vi "VideoWriter GetBackendName.vi"(8 "error in (no error)":errorcluster, 11 "VideoWriter in":refnum<class "VideoWriter.lvclass">) -> (0 "error out":errorcluster, 2 "BackendName":string, 3 "VideoWriter out":refnum<class "VideoWriter.lvclass">)   [LabVIEW 2020, in "OpenLvVision_OpenCv.lvlib" / "VideoWriter.lvclass"]
doc: "Returns used backend API name."
uses:
  VideoWriter.lvclass
  C:/Users/lukas/Downloads/OpenLvVision_OpenCv/SourceCode/LabView/OpenLvVision_OpenCv/_LvHelpers/EdvrObject/EdvrObject.lvclass
  _LvHelpers/EdvrObject/EdvrObject.lvclass/EdvrObject.ctl
  OpenLvVision_OpenCv.lvlib
  _LvHelpers/EdvrObject/EdvrObject.lvclass
  Dlls/OlvOpenCvWrapper.dll
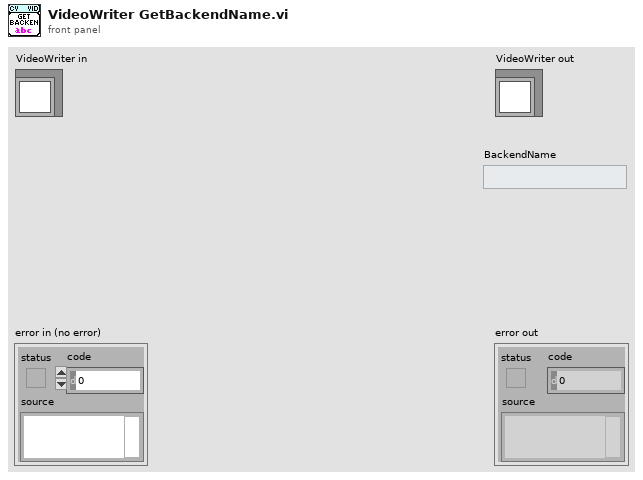
[diagram p1: front panel]
types:
  T1 = typedef "OpenLvVision_OpenCv.lvlib/EdvrObject.lvclass/Edvr.ctl" = refnum<data-value>
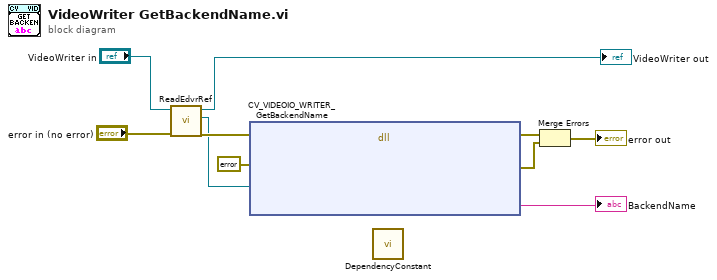
[diagram p0: block diagram]
diagram:
  n1 = call "ReadEdvrRef.vi"("error in (no error)"="error in (no error)", "EdvrObject in"="VideoWriter in") -> ("error out"=w9:errorcluster, "Edvr"=w8:T1, "EdvrObject out"=→"VideoWriter out":refnum<class "VideoWriter.lvclass">)  [unwired: 7 in]
  n2 = dll-call lib="C:/Users/lukas/Downloads/OpenLvVision_OpenCv/SourceCode/LabView/OpenLvVision_OpenCv/Dlls/OlvOpenCvWrapper.dll" fn="CV_VIDEOIO_WRITER_GetBackendName"(error in=w9, "Error"=errorcluster {"status"=FALSE, "code"=0, "source"=""} ("error out"), "edvrRef"=w8) -> (error out=w7:errorcluster, "Error"=w4:errorcluster, "resultHandle"=→"BackendName":string)  [unwired: 5 in, 1 out]
  n3 = call "DependencyConstant.vi"() -> ()  [unwired: 12 in]
  n4 = Merge Errors(w7, w4) -> (→"error out":errorcluster)
